vi "Read Totalizer Units and Decimals.vi"(7 "Unit ID (A)":string="A", 8 "error in":errorcluster, 10 "Software Version":u8, 11 "VISA Session In":refnum<visa-resource-name>="Alicat") -> (0 "error out":errorcluster, 1 "Totalizer Units":string, 2 "Totalizer":T2(ring), 3 "VISA Session Out":refnum<visa-resource-name>, 4 "Totalizer decimal places":i32)   [LabVIEW 2020]
doc: "Returns the variable of the totalizer (if applicable), the totalizer units (as a string), and the number of decimals of the totalizer data."
uses:
  <vilib>/Instr/_visa.llb/VISA Flush IO Buffer Mask.ctl
panel:
  out "Total Volume Units":u16(ring)=1 items=["Default"=0, "Unknown"=1, "uL"=2, "mL"=3, "L"=4, "US GAL"=5, "cm3"=6, "m3"=7, "in3"=8, "ft3"=9, "uP"=61]
  out "Total Mass Units":u16(ring)=1 items=["Default"=0, "Unknown"=1, "SuL"=2, "SmL"=3, "SL"=4, "Scm3"=6, "Sm3"=7, "Sin3"=8, "Sft3"=9, "kSft3"=10, "NuL"=32, "NmL"=33, "NL"=34, "Ncm3"=35, "Nm3"=36, "mg"=64, "g"=65, "kg"=66, "oz"=67, "lb"=68]
  out "Totalizer Units":T1(ring)
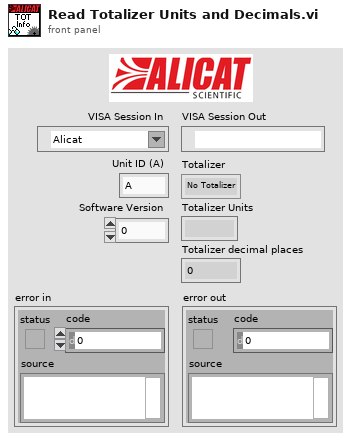
[diagram p1: front panel]
types:
  T1 = enum8{"CC", "uL", "L", "CI", "CF", "CM", "GAL", "mL", "uP", "Lbs", "N/A", "unknown (11)", "unknown (12)", "SCC", "SuL", "SL", "SCI", "SCF", "NCM", "Grams", "Kg", "lbs", "mg", "SCM", "smL", "KSCF"}
  T2 = enum8{"No Totalizer", "Mass Flow", "Volumetric Flow"}
  T3 = typedef "VISA Flush IO Buffer Mask.ctl" = u16
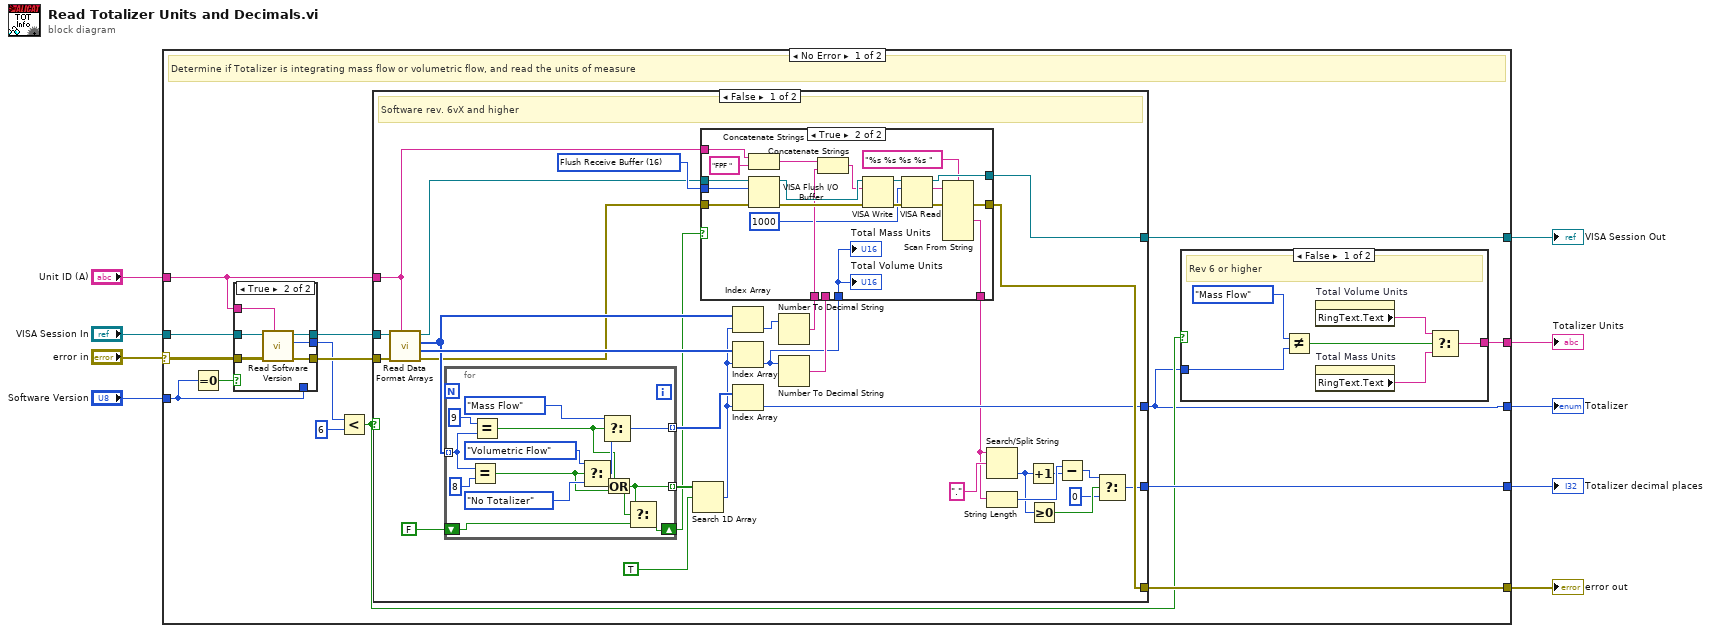
[diagram p0: block diagram]
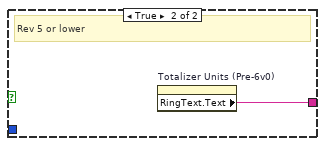
[diagram p2: hidden frame]
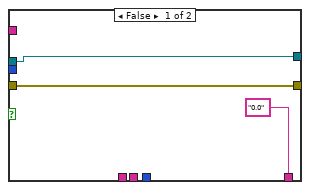
[diagram p4: hidden frame]
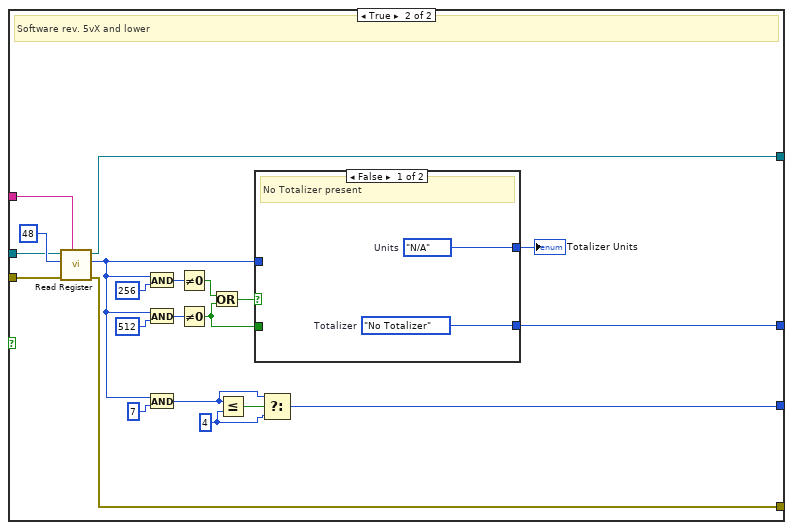
[diagram p5: hidden frame]
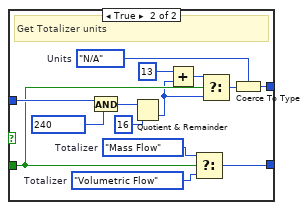
[diagram p6: hidden frame]
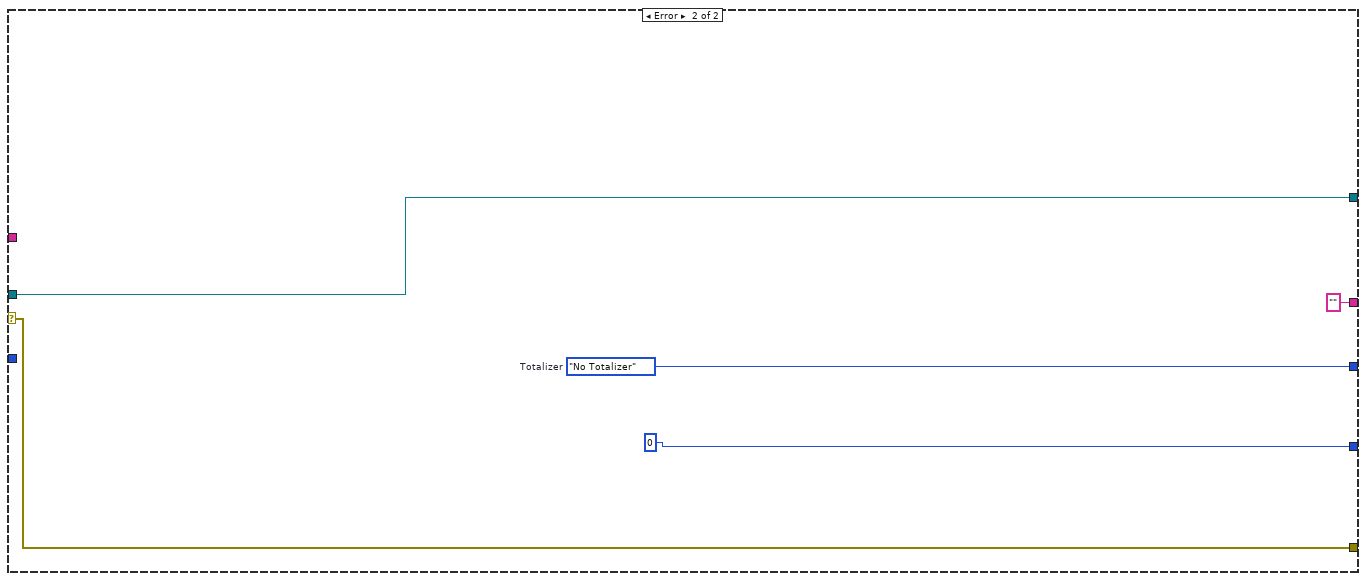
[diagram p7: hidden frame]
diagram:
  n1 = case shown="No Error" "error in" {
    selector: "error in" -> [w17 w148]
    tunnel: "VISA Session In" -> [w18 w147]
    tunnel: [w24 w147] -> w8
    tunnel: "Unit ID (A)" -> [w19 _]
    tunnel: [w23 w148] -> w6
    tunnel: [w11 w146] -> w4
    tunnel: [w22 0] -> w3
    tunnel: "Software Version" -> [w20 _]
    tunnel: [w10 "" ("RingText.Text")] -> w1
    frame No Error {
      # "Determine if Totalizer is integrating mass flow or volumetric flow, and read the units of measure"
      n2 = Equal To 0?(x=w20) -> (x = 0?=w21:bool)
      n3 = case shown="True" w21 {
        tunnel: w17 -> [w33 w40]
        tunnel: w18 -> [w32 w39]
        tunnel: w19 -> [_ w38]
        tunnel: [w33 w37] -> w16
        tunnel: [w32 w36] -> w15
        tunnel: [w34 w35] -> w13
        tunnel: w20 -> [w34 _]
        frame False {
        }
        frame True {
          n4 = call "Read Software Version.vi"("Unit ID (A)"=w38, "error in"=w40, "VISA Session In"=w39) -> ("error out"=w37:errorcluster, "Software Version"=w35:u8, "VISA Session Out"=w36:refnum<visa-resource-name>)  [unwired: 6 in]
        }
      }
      n5 = Less?(x=w13, y=u8 6) -> (x < y?=w12:bool)
      n6 = case shown="False" w12 {
        tunnel: w15 -> [w70 w126]
        tunnel: [w56 w125] -> w24
        tunnel: w19 -> [w63 w124]
        tunnel: [w54 w123] -> w23
        tunnel: w16 -> [w69 w115]
        tunnel: [w51 w114] -> w11
        tunnel: [w41 w108] -> w22
        frame False {
          w65 = T3 16 items=["Flush Receive Buffer"=16, "Write Transmit Buffer to Device"=32, "Flush Receive Buffer (No I/O)"=64, "Flush Transmit Buffer"=128] ("Mask")
          # "Software rev. 6vX and higher"
          n7 = call "Read Data Format Arrays.vi"("Unit ID (A)"=w63, "error in (no error)"=w69, "VISA Session In"=w70) -> ("error out"=w55:errorcluster, "Units Array"=w62:u16[], "Data Type Array"=w61:u16[], "VISA Session Out"=w64:refnum<visa-resource-name>)  [unwired: 5 in]
          n8 = for {
            tunnel: w61 -> [w105] mode=indexing
            tunnel: [w99] -> w66 mode=indexing
            tunnel: [w95] -> w68 mode=indexing
            shift-right: [w96] -> w53
            shift-left: FALSE ("element") -> [w94]
            n9 = Equal?(x=w105, y=u16 8 ("x")) -> (x = y?=w97:bool)
            n10 = Equal?(x=u16 9, y=w105) -> (x = y?=w98:bool)
            n11 = Select(t=T2."Volumetric Flow" ("Totalizer"), s=w97, f=T2."No Totalizer" ("Totalizer")) -> (s? t:f=w102:T2)
            n12 = Select(t=T2."Mass Flow" ("Totalizer"), s=w98, f=w102) -> (s? t:f=w99:T2)
            n13 = Or(x=w98, y=w97) -> (x .or. y?=w95:bool)
            n14 = Select(t=w95, s=w95, f=w94) -> (s? t:f=w96:bool)
          }
          n15 = Search 1D Array(1D array=w68, element=TRUE) -> (index of element=w60:i32)  [unwired: 1 in]
          n16 = Index Array(array=w61, index=w60) -> (element=w59:u16)
          n17 = Index Array(array=w62, index=w60) -> (element=w50:u16)
          n18 = Index Array(array=w66, index=w60) -> (element=w51:T2)
          n19 = Number To Decimal String(number=w59) -> (decimal integer string=w58:string)  [unwired: 1 in]
          n20 = Number To Decimal String(number=w50) -> (decimal integer string=w57:string)  [unwired: 1 in]
          n21 = case shown="True" w53 {
            tunnel: w65 -> [_ w93]
            tunnel: w64 -> [w73 w89]
            tunnel: w63 -> [_ w88]
            tunnel: w58 -> [_ w85]
            tunnel: w57 -> [_ _]
            tunnel: [w73 w82] -> w56
            tunnel: w55 -> [w72 w81]
            tunnel: [w72 w77] -> w54
            tunnel: ["0.0" w76] -> w42
            tunnel: w50 -> [_ w75]
            frame False {
            }
            frame True {
              n22 = Concatenate Strings(w88, "FPF " ("string")) -> (w87:string)
              n23 = VISA Flush I/O Buffer(VISA resource name=w89, mask (16)=w93, error in (no error)=w81) -> (VISA resource name out=w92:refnum<visa-resource-name>, error out=w91:errorcluster)
              n24 = Concatenate Strings(w87, w85) -> (w86:string)
              n25 = VISA Write(VISA resource name=w92, write buffer=w86, error in (no error)=w91) -> (VISA resource name out=w83:refnum<visa-resource-name>, error out=w84:errorcluster)  [unwired: 1 out]
              n26 = VISA Read(VISA resource name=w83, byte count=u32 1000, error in (no error)=w84) -> (VISA resource name out=w82:refnum<visa-resource-name>, read buffer=w80:string, error out=w78:errorcluster)  [unwired: 1 out]
              n27 = Scan From String(format string="%s %s %s %s ", input string=w80, error in=w78) -> (error out=w77:errorcluster, output 2=w76:string)  [unwired: 8 in, 2 out]
              "Total Mass Units" <- w75
              "Total Volume Units" <- w75
            }
          }
          n28 = Search/Split String(string=w42, search string/char (-)="." ("regular expression")) -> (offset of match=w46:i32)  [unwired: 1 in, 2 out]
          n29 = String Length(string=w42) -> (length=w49:i32)
          n30 = Increment(x=w46) -> (x+1=w47:i32)
          n31 = Greater Or Equal To 0?(x=w46) -> (x >= 0?=w44:bool)
          n32 = Subtract(x=w49, y=w47) -> (x-y=w45:i32)
          n33 = Select(t=w45, s=w44, f=0) -> (s? t:f=w41:i32)
        }
        frame True {
          w109 = 4
          # "Software rev. 5vX and lower"
          n34 = call "Read Register.vi"("Unit ID (A)"=w124, "error in"=w115, "Register address"=u16 48 ("register"), "VISA Session In"=w126) -> ("error out"=w123:errorcluster, "Register Value (I32)"=w112:i32, "VISA Session Out"=w125:refnum<visa-resource-name>)  [unwired: 5 in]
          n35 = And(x=w112, y=256) -> (x .and. y?=w122:i32)
          n36 = And(x=w112, y=512) -> (x .and. y?=w120:i32)
          n37 = And(x=w112, y=7) -> (x .and. y?=w110:i32)
          n38 = Not Equal To 0?(x=w122) -> (x != 0?=w118:bool)
          n39 = Not Equal To 0?(x=w120) -> (x != 0?=w116:bool)
          n40 = Or(x=w118, y=w116) -> (x .or. y?=w117:bool)
          n41 = Less Or Equal?(x=w110, y=w109) -> (x <= y?=w111:bool)
          n42 = case shown="False" w117 {
            tunnel: [w129 w130] -> w107
            tunnel: [w128 w141] -> w114
            tunnel: w116 -> [_ w136]
            tunnel: w112 -> [_ w140]
            frame False {
              w128 = T2."No Totalizer"  # Totalizer
              w129 = T1."N/A"  # Units
              # "No Totalizer present"
            }
            frame True {
              w131 = T1."N/A"  # Units
              w143 = T2."Mass Flow"  # Totalizer
              w142 = T2."Volumetric Flow"  # Totalizer
              # "Get Totalizer units"
              n43 = And(x=w140, y=240 ("Numeric 2")) -> (x .and. y?=w138:i32)
              n44 = Quotient & Remainder(x=w138, y=16) -> (floor(x/y)=w134:i32)  [unwired: 1 out]
              n45 = Add(x=13, y=w134) -> (x+y=w135:i32)
              n46 = Select(t=w143, s=w136, f=w142) -> (s? t:f=w141:T2)
              n47 = Select(t=w135, s=w136, f=w134) -> (s? t:f=w132:i32)
              n48 = Coerce To Type(0:w132, 1:w131) -> (2:w130:T1)
            }
          }
          "Totalizer Units" <- w107
          n49 = Select(t=w110, s=w111, f=w109) -> (s? t:f=w108:i32)
        }
      }
      n50 = case shown="False" w12 {
        tunnel: w11 -> [w25 _]
        tunnel: [w27 w31] -> w10
        frame False {
          # "Rev 6 or higher"
          n51 = Not Equal?(x=T2."Mass Flow" ("Totalizer"), y=w25) -> (x != y?=w26:bool)
          n52 = property on="Total Volume Units" class="Ring (strict)"() -> ("RingText.Text"=w29:string)  [unwired: 2 in, 2 out]
          n53 = property on="Total Mass Units" class="Ring (strict)"() -> ("RingText.Text"=w28:string)  [unwired: 2 in, 2 out]
          n54 = Select(t=w29, s=w26, f=w28) -> (s? t:f=w27:string)
        }
        frame True {
          # "Rev 5 or lower"
          n55 = property on="Totalizer Units (Pre-6v0)" class="Enum (strict)"() -> ("RingText.Text"=w31:string)  [unwired: 2 in, 2 out]
        }
      }
    }
    frame Error {
      w146 = T2."No Totalizer"  # Totalizer
    }
  }
  "error out" <- w6
  "VISA Session Out" <- w8
  "Totalizer" <- w4
  "Totalizer decimal places" <- w3
  "Totalizer Units" <- w1
